vi "sub9choice.vi"(8 "error in":errorcluster, 10 "Detector Start Pin":u8, 11 "Arduino Resource":T1={"VISA resource"="", "Board Type"=enum."Uno", "Connection Type"=enum."USB / Serial", "Bytes Per Packet (15)"=15}) -> (0 "error out":errorcluster, 2 "Ouput":dbl, 3 "Arduino Resource 2":T1={"VISA resource"="", "Board Type"=enum."Uno", "Connection Type"=enum."USB / Serial", "Bytes Per Packet (15)"=15})   [LabVIEW 2016]
uses:
  <vilib>/LabVIEW Interface for Arduino/Type Defs/Arduino Resource.ctl
  <vilib>/LabVIEW Interface for Arduino/Type Defs/Board Type.ctl
  <vilib>/LabVIEW Interface for Arduino/LabVIEW Interface for Arduino.lvlib
panel:
  out "Boolean 6":bool
  out "Boolean 7":bool
  out "Boolean 8":bool
  out "Boolean 9":bool
  out "Boolean 1":bool
  out "Boolean 2":bool
  out "Boolean 3":bool
  out "Boolean 4":bool
  out "Boolean 5":bool
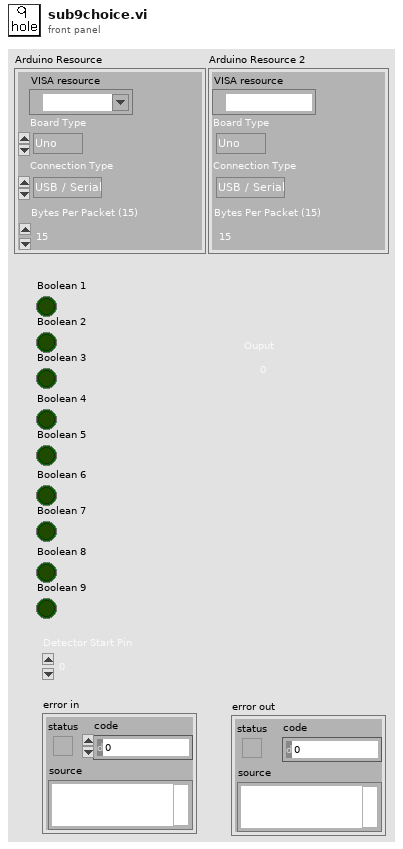
[diagram p1: front panel]
types:
  T1 = typedef "LabVIEW Interface for Arduino.lvlib/Arduino Resource.ctl" = cluster{"VISA resource":refnum<visa-resource-name>, "Board Type":T2, "Connection Type":enum8{"USB / Serial"}, "Bytes Per Packet (15)":u8}
  T2 = typedef "LabVIEW Interface for Arduino.lvlib/Board Type.ctl" = enum16{"Uno", "Dimuelanove w/Atmega 328", "Mega 2560"}
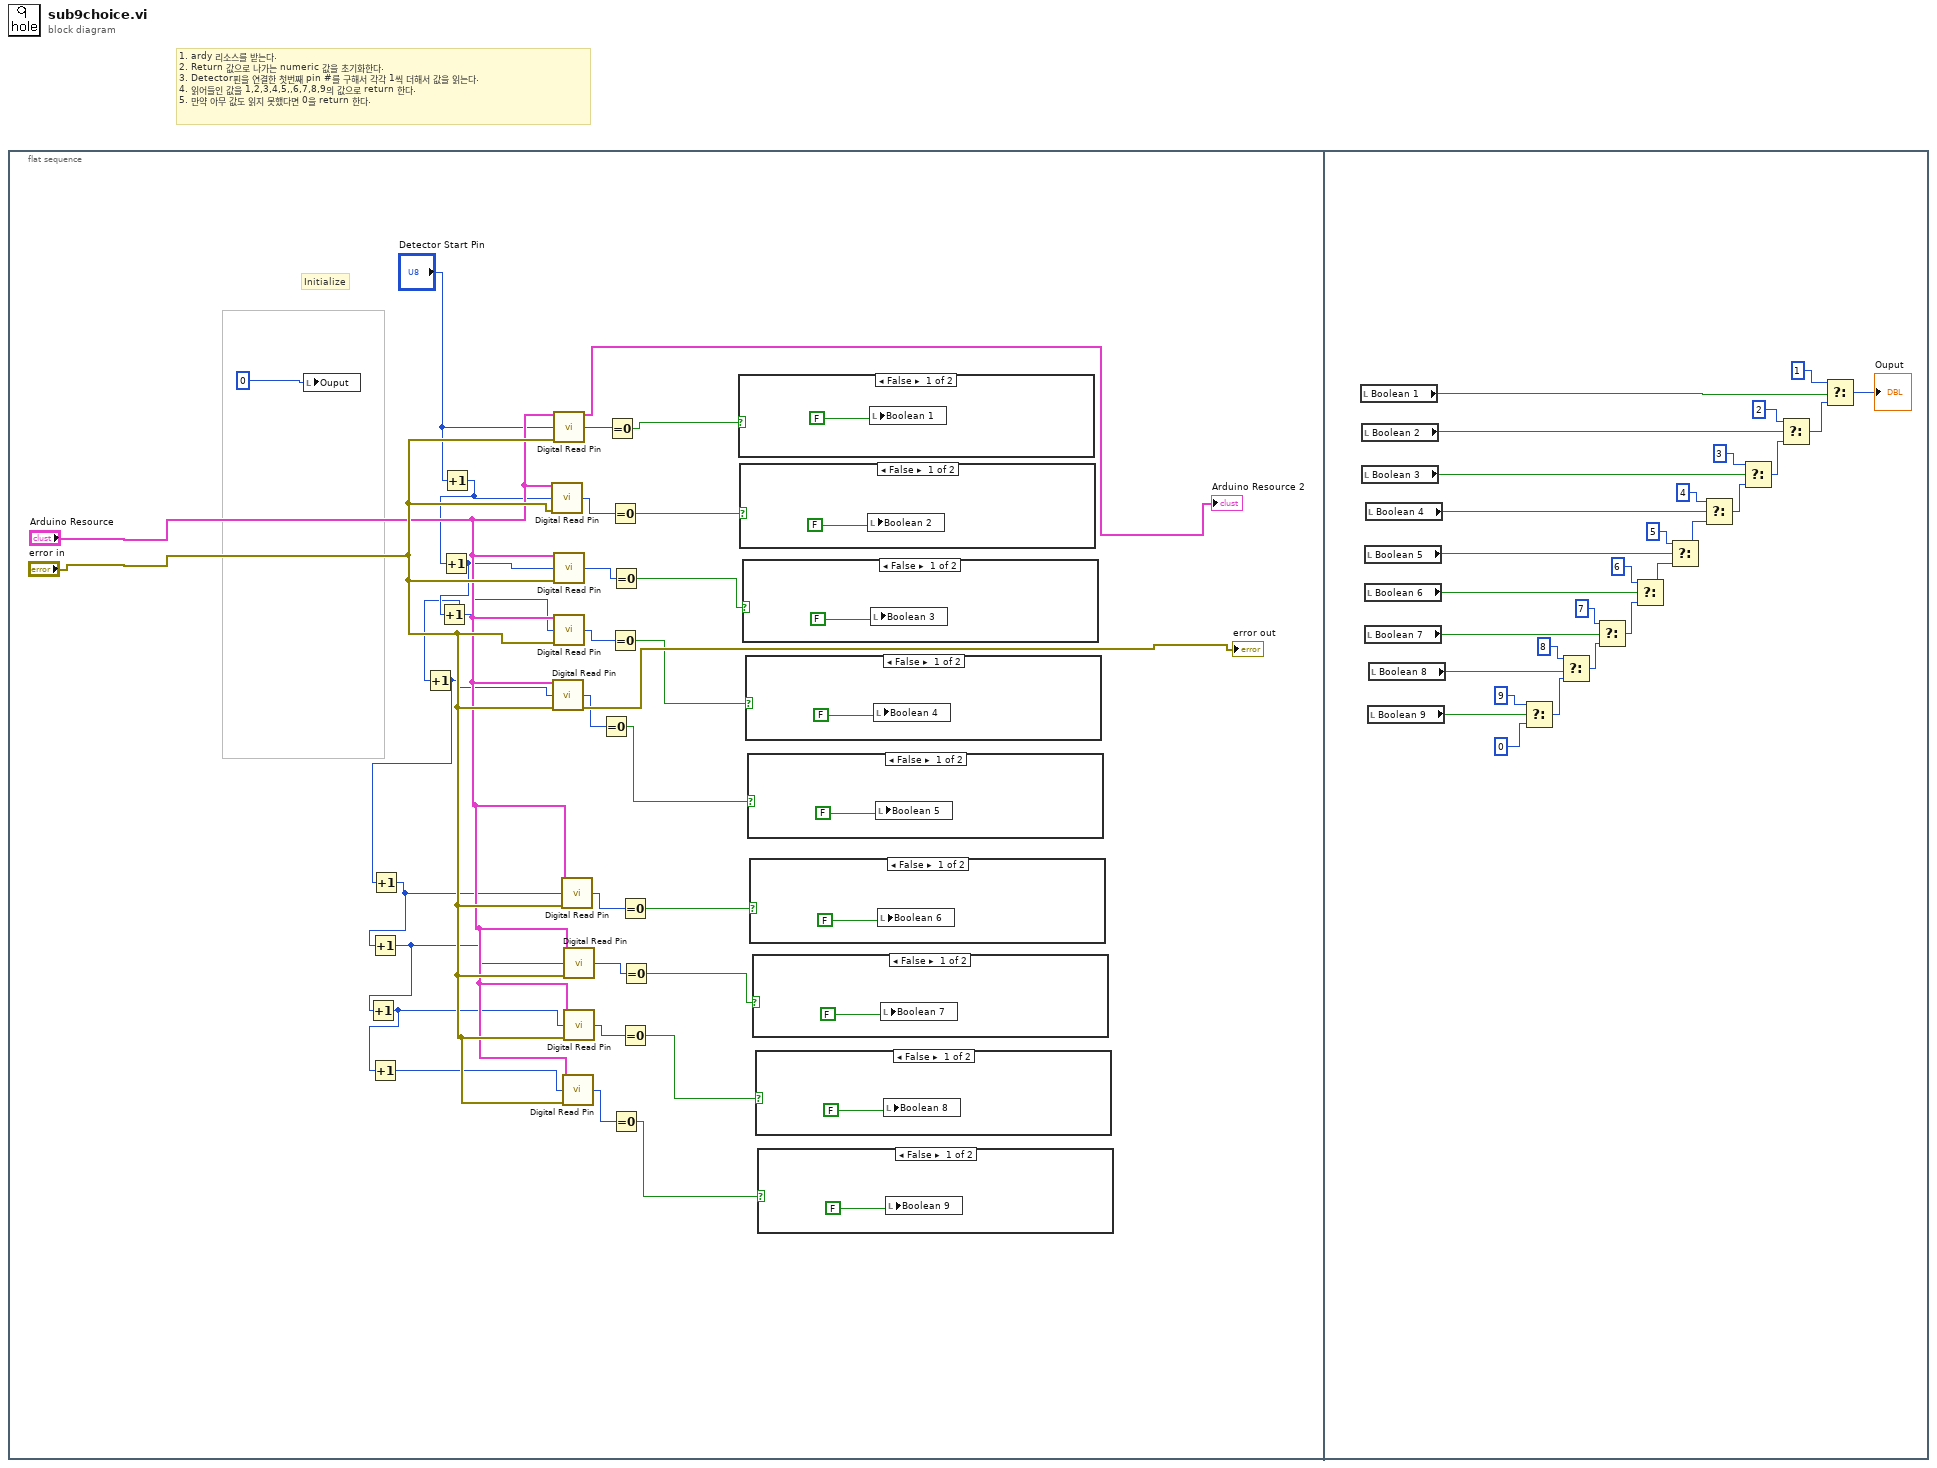
[diagram p0: block diagram]
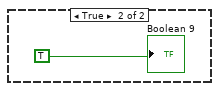
[diagram p2: hidden frame]
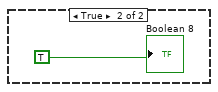
[diagram p3: hidden frame]
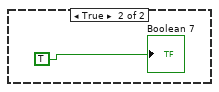
[diagram p4: hidden frame]
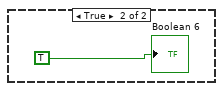
[diagram p5: hidden frame]
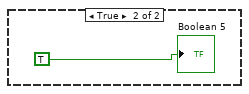
[diagram p6: hidden frame]
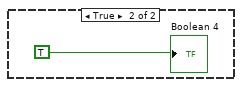
[diagram p7: hidden frame]
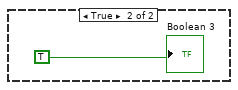
[diagram p8: hidden frame]
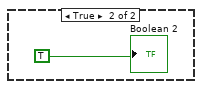
[diagram p9: hidden frame]
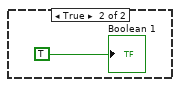
[diagram p10: hidden frame]
diagram:
  # "1. ardy 리소스를 받는다. \n2. Return 값으로 나가는 numeric 값을 초기화한다.\n3. Detector핀을 연결한 첫번째 pin #를 구해서 각각 1씩 더해서 값을 읽는다.\n4. 읽어들인 값을 1,2,3,4,5,,6,7,8,9의 값으로 return 한다. \n5. 만약 아무 값도 읽지 못했다면 0을 return 한다."
  n1 = flat-sequence {
    frame #0 {
      # "Initialize"
      n2 = local write "Ouput"(0) -> ()
      n3 = Increment(x="Detector Start Pin") -> (x+1=w8:u8)
      n4 = Increment(x=w8) -> (x+1=w7:u8)
      n5 = Increment(x=w7) -> (x+1=w6:u8)
      n6 = Increment(x=w6) -> (x+1=w5:u8)
      n7 = Increment(x=w5) -> (x+1=w4:u8)
      n8 = Increment(x=w4) -> (x+1=w3:u8)
      n9 = Increment(x=w3) -> (x+1=w2:u8)
      n10 = Increment(x=w2) -> (x+1=w1:u8)
      n11 = call <vilib>:"Digital Read Pin.vi"("Arduino Resource"="Arduino Resource", "Digital I/O Pin (0)"=w8, "error in"="error in") -> ("Value"=w23:u8)  [unwired: 10 in, 2 out]
      n12 = call <vilib>:"Digital Read Pin.vi"("Arduino Resource"="Arduino Resource", "Digital I/O Pin (0)"=w5, "error in"="error in") -> ("Value"=w20:u8, "error out"=→"error out":errorcluster)  [unwired: 10 in, 1 out]
      n13 = call <vilib>:"Digital Read Pin.vi"("Arduino Resource"="Arduino Resource", "Digital I/O Pin (0)"="Detector Start Pin", "error in"="error in") -> ("Arduino Resource"=→"Arduino Resource 2":T1, "Value"=w24:u8)  [unwired: 10 in, 1 out]
      n14 = call <vilib>:"Digital Read Pin.vi"("Arduino Resource"="Arduino Resource", "Digital I/O Pin (0)"=w7, "error in"="error in") -> ("Value"=w22:u8)  [unwired: 10 in, 2 out]
      n15 = call <vilib>:"Digital Read Pin.vi"("Arduino Resource"="Arduino Resource", "Digital I/O Pin (0)"=w6, "error in"="error in") -> ("Value"=w21:u8)  [unwired: 10 in, 2 out]
      n16 = call <vilib>:"Digital Read Pin.vi"("Arduino Resource"="Arduino Resource", "Digital I/O Pin (0)"=w4, "error in"="error in") -> ("Value"=w16:u8)  [unwired: 10 in, 2 out]
      n17 = call <vilib>:"Digital Read Pin.vi"("Arduino Resource"="Arduino Resource", "Digital I/O Pin (0)"=w1, "error in"="error in") -> ("Value"=w19:u8)  [unwired: 10 in, 2 out]
      n18 = call <vilib>:"Digital Read Pin.vi"("Arduino Resource"="Arduino Resource", "Digital I/O Pin (0)"=w3, "error in"="error in") -> ("Value"=w17:u8)  [unwired: 10 in, 2 out]
      n19 = call <vilib>:"Digital Read Pin.vi"("Arduino Resource"="Arduino Resource", "Digital I/O Pin (0)"=w2, "error in"="error in") -> ("Value"=w18:u8)  [unwired: 10 in, 2 out]
      n20 = Equal To 0?(x=w20) -> (x = 0?=w25:bool)
      n21 = Equal To 0?(x=w24) -> (x = 0?=w29:bool)
      n22 = Equal To 0?(x=w23) -> (x = 0?=w28:bool)
      n23 = Equal To 0?(x=w21) -> (x = 0?=w26:bool)
      n24 = Equal To 0?(x=w22) -> (x = 0?=w27:bool)
      n25 = Equal To 0?(x=w19) -> (x = 0?=w15:bool)
      n26 = Equal To 0?(x=w16) -> (x = 0?=w12:bool)
      n27 = Equal To 0?(x=w18) -> (x = 0?=w14:bool)
      n28 = Equal To 0?(x=w17) -> (x = 0?=w13:bool)
      n29 = case shown="False" w29 {
        frame False {
          n30 = local write "Boolean 1"(FALSE) -> ()
        }
        frame True {
          "Boolean 1" <- TRUE
        }
      }
      n31 = case shown="False" w28 {
        frame False {
          n32 = local write "Boolean 2"(FALSE) -> ()
        }
        frame True {
          "Boolean 2" <- TRUE
        }
      }
      n33 = case shown="False" w27 {
        frame False {
          n34 = local write "Boolean 3"(FALSE) -> ()
        }
        frame True {
          "Boolean 3" <- TRUE
        }
      }
      n35 = case shown="False" w26 {
        frame False {
          n36 = local write "Boolean 4"(FALSE) -> ()
        }
        frame True {
          "Boolean 4" <- TRUE
        }
      }
      n37 = case shown="False" w25 {
        frame False {
          n38 = local write "Boolean 5"(FALSE) -> ()
        }
        frame True {
          "Boolean 5" <- TRUE
        }
      }
      n39 = case shown="False" w12 {
        frame False {
          n40 = local write "Boolean 6"(FALSE) -> ()
        }
        frame True {
          "Boolean 6" <- TRUE
        }
      }
      n41 = case shown="False" w13 {
        frame False {
          n42 = local write "Boolean 7"(FALSE) -> ()
        }
        frame True {
          "Boolean 7" <- TRUE
        }
      }
      n43 = case shown="False" w14 {
        frame False {
          n44 = local write "Boolean 8"(FALSE) -> ()
        }
        frame True {
          "Boolean 8" <- TRUE
        }
      }
      n45 = case shown="False" w15 {
        frame False {
          n46 = local write "Boolean 9"(FALSE) -> ()
        }
        frame True {
          "Boolean 9" <- TRUE
        }
      }
    }
    frame #1 {
      n47 = local read "Boolean 1"() -> (w78:bool)
      n48 = local read "Boolean 2"() -> (w76:bool)
      n49 = local read "Boolean 3"() -> (w75:bool)
      n50 = local read "Boolean 5"() -> (w70:bool)
      n51 = local read "Boolean 6"() -> (w61:bool)
      n52 = local read "Boolean 7"() -> (w60:bool)
      n53 = local read "Boolean 4"() -> (w72:bool)
      n54 = local read "Boolean 9"() -> (w53:bool)
      n55 = local read "Boolean 8"() -> (w55:bool)
      n56 = Select(t=9, s=w53, f=0) -> (s? t:f=w51:i32)
      n57 = Select(t=8, s=w55, f=w51) -> (s? t:f=w57:i32)
      n58 = Select(t=7, s=w60, f=w57) -> (s? t:f=w59:i32)
      n59 = Select(t=6, s=w61, f=w59) -> (s? t:f=w62:i32)
      n60 = Select(t=5, s=w70, f=w62) -> (s? t:f=w71:i32)
      n61 = Select(t=4, s=w72, f=w71) -> (s? t:f=w73:i32)
      n62 = Select(t=3, s=w75, f=w73) -> (s? t:f=w74:i32)
      n63 = Select(t=2, s=w76, f=w74) -> (s? t:f=w77:i32)
      n64 = Select(t=1, s=w78, f=w77) -> (s? t:f=→"Ouput":i32)
    }
  }
